vi "SPI Write Read.vi"(4 "CS Logic Level":T1, 6 "CS Pin (10)":u8=10, 7 "SPI Frame Size (1)":u8=1, 8 "Error In":errorcluster, 9 "Data":u8[](array[numeric]), 10 "SPI Channel":u8, 11 "LINX Device Config":T2) -> (0 "Error Out":errorcluster, 1 "Read Data":u8[](array[numeric]), 3 "LINX Device Config":T2)   [LabVIEW 2013, in "LVH-LINX.lvlib" / "Device.lvlib"]
doc: "Write/Read the specified SPI channel."
uses:
  <vilib>/LabVIEW Hacker/LINX/Private/Device/Device.lvlib
  <vilib>/LabVIEW Hacker/LINX/Private/Device/Type Defs/LINX Device Config.ctl
  <vilib>/LabVIEW Hacker/LINX/Private/Type Defs/Interface.ctl
  <vilib>/LabVIEW Hacker/LINX/Private/Device/Type Defs/TCP Config.ctl
  <vilib>/LabVIEW Hacker/LINX/Private/Type Defs/Device Family.ctl
  <vilib>/LabVIEW Hacker/LINX/Private/Type Defs/Peripherals/SPI/SPI CS Logic Level.ctl
  <vilib>/LabVIEW Hacker/LINX/Private/Type Defs/Error Type.ctl
  <vilib>/LabVIEW Hacker/LINX/LVH-LINX.lvlib
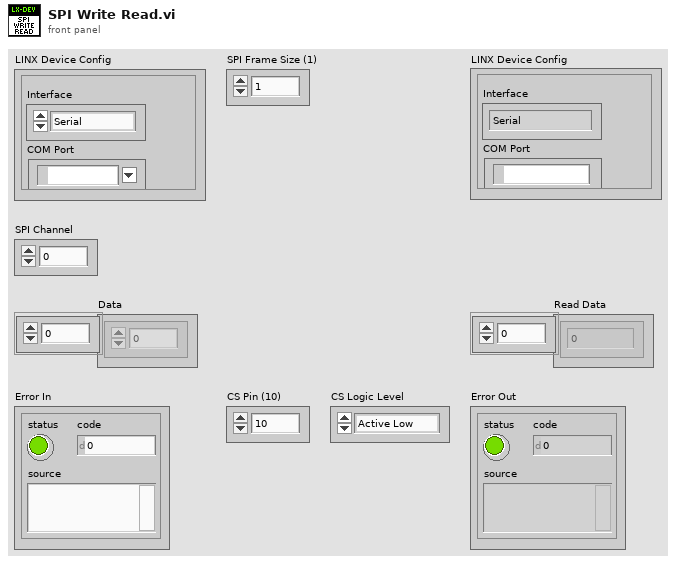
[diagram p1: front panel]
types:
  T1 = typedef "LVH-LINX.lvlib/SPI CS Logic Level.ctl" = enum8{"Active Low", "Active High"}
  T2 = typedef "LVH-LINX.lvlib/Device.lvlib/LINX Device Config.ctl" = cluster{"Interface":T3, "COM Port":refnum<visa-resource-name>, "TCP Configuration":T4, "Device Family":T5, "Device ID":u8, "Device Name":string, "TCP Ref":refnum<k5>}
  T3 = typedef "LVH-LINX.lvlib/Interface.ctl" = enum16{"Serial", "TCP"}
  T4 = typedef "LVH-LINX.lvlib/Device.lvlib/TCP Config.ctl" = cluster{"IP Address":string, "Port":u16}
  T5 = typedef "LVH-LINX.lvlib/Device Family.ctl" = enum8{"National Instruments", "Digilent", "Arduino"}
  T6 = typedef "LVH-LINX.lvlib/Error Type.ctl" = enum16{"Unknown", "Timeout", "Corrupt Return Packet", "Unable To Connect", "Command Not Supported", "Channel DNE", "Invalid COM Config"}
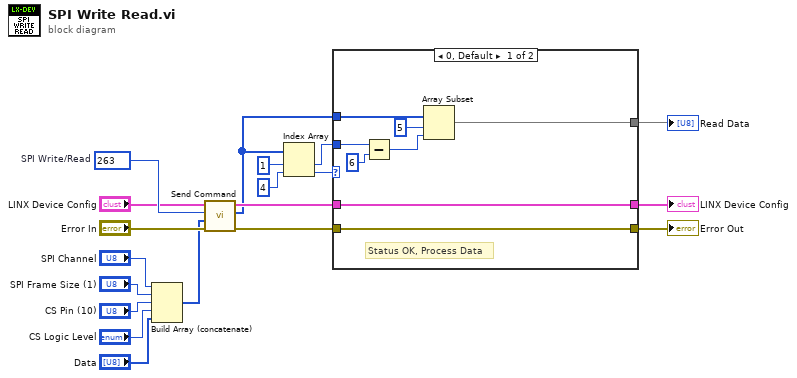
[diagram p0: block diagram]
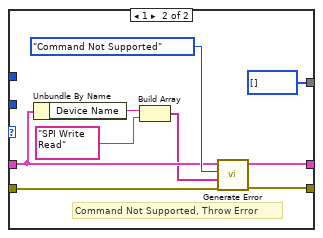
[diagram p2: hidden frame]
diagram:
  w18 = u16 263  # SPI Write/Read
  n1 = Build Array (concatenate)("SPI Channel", "SPI Frame Size (1)", "CS Pin (10)", "CS Logic Level", "Data") -> (w11:u8[])
  n2 = call <vilib>:"Send Command.vi"("Error In"="Error In", "ARGS"=w11, "CMD"=w18, "LINX Device Config"="LINX Device Config") -> ("Error Out"=w13:errorcluster, "Response"=w10:u8[], "LINX Device Config"=w15:T2)  [unwired: 4 in, 1 out]
  n3 = Index Array(array=w10, index #1=1 ("index"), index #2=4 ("index")) -> (element #1=w6:u8, element #2=w7:u8)
  n4 = case shown="0, Default" w7 {
    tunnel: [w27 w34] -> w16
    tunnel: w15 -> [w27 w30]
    tunnel: [w26 w35] -> w14
    tunnel: w13 -> [w26 w36]
    tunnel: w10 -> [w25 _]
    tunnel: w6 -> [w24 _]
    tunnel: [w20 u8[] []] -> w5
    frame 0, Default {
      # "Status OK, Process Data"
      n5 = Subtract(x=w24, y=u8 6) -> (x-y=w22:u8)
      n6 = Array Subset(array=w25, index=5, length=w22) -> (w20:u8[])
    }
    frame 1 {
      # "Command Not Supported, Throw Error"
      n7 = Unbundle By Name(w30) -> ("Device Name"=w32:string)
      n8 = Build Array(w32, "SPI Write Read") -> (w29:string[])
      n9 = call <vilib>:"Generate Error.vi"("Error In"=w36, "Arguments"=w29, "Error Type"=Error_Type."Command Not Supported", "LINX Device Config"=w30) -> ("Error Out"=w35:errorcluster, "LINX Device Config"=w34:T2)  [unwired: 6 in]
    }
  }
  "Error Out" <- w14
  "LINX Device Config" <- w16
  "Read Data" <- w5
